vi "motor_log.vi"() -> ()   [LabVIEW 2011]
uses:
  <vilib>/addons/database/Auxilliary.llb/DB Tools Format Datetime String (Time Stamp).vi
  <vilib>/addons/database/Connection.llb/DB Tools Open Connec (String).vi
  <vilib>/addons/database/NI_Database_API.lvlib
  Program Files (x86)/National Instruments/LabVIEW 2011/resource/objmgr/daqmx.rc
panel:
  out "Channels":refnum<k21>[](array[refnum])
  out "decimal integer string":string
  out "Array":dbl[](array[numeric])
  out "Degrees":u32
  out "Boolean 2":bool
  out "Steps":u32
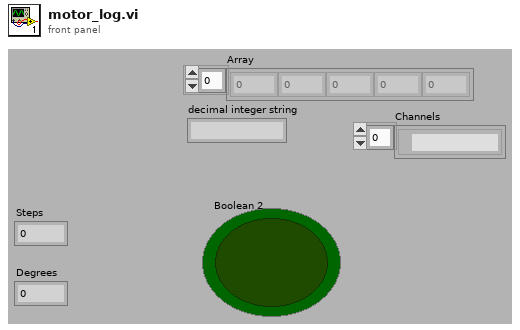
[diagram p1: front panel]
types:
  T1 = typedef "NI_Database_API.lvlib/Conn ObjectReference.ctl" = refnum<k1>
  T2 = cluster{"Array[0]":dbl, "Array[1]":dbl, "Array[2]":dbl, "Array[3]":dbl, "Array[4]":dbl, "Array[5]":dbl, "Array[6]":dbl, "Array[7]":dbl, "Array[8]":dbl}
  T3 = cluster{"date/time string":string, dbl, "Array":cluster{"Array[0]":dbl, "Array[1]":dbl, "Array[2]":dbl, "Array[3]":dbl, "Array[4]":dbl, "Array[5]":dbl, "Array[6]":dbl, "Array[7]":dbl, "Array[8]":dbl}}
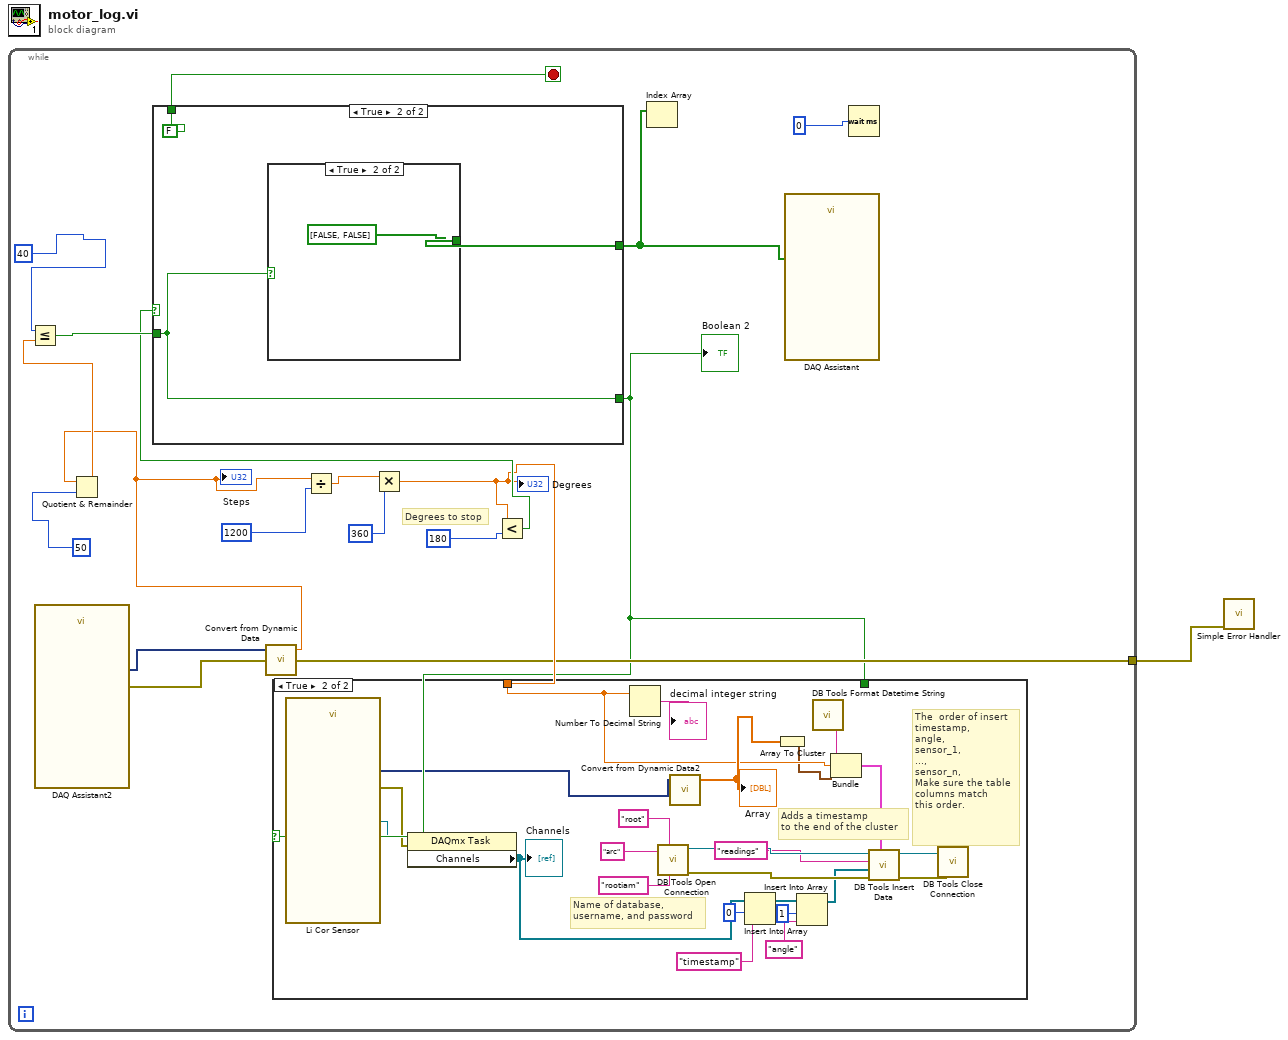
[diagram p0: block diagram]
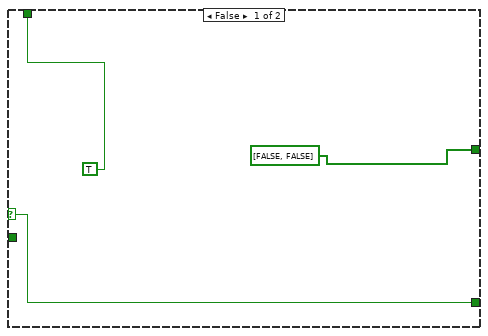
[diagram p3: hidden frame]
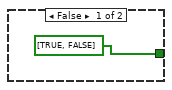
[diagram p4: hidden frame]
diagram:
  n1 = while {
    tunnel: [w5] -> w1
    stop <- w10 stop-if-true
    # "Degrees to stop"
    n2 = call "DAQ Assistant2"() -> ("data"=w6:dynamicdata, "error out"=w5:errorcluster)  [unwired: 16 in, 2 out]
    n3 = call "Convert from Dynamic Data"("Dynamic Data Type"=w6) -> ("Scalar"=w8:dbl)  [unwired: 3 in]
    "Steps" <- w8
    n4 = Quotient & Remainder(x=w8, y=50) -> (x-y*floor(x/y)=w12:dbl)  [unwired: 1 out]
    n5 = Less Or Equal?(x=40, y=w12) -> (x <= y?=w18:bool)
    n6 = Divide(x=w8, y=1200) -> (x/y=w16:dbl)
    n7 = Multiply(x=w16, y=360) -> (x*y=w7:dbl)
    "Degrees" <- w7
    n8 = Less?(x=w7, y=180) -> (x < y?=w11:bool)
    n9 = case shown="True" w11 {
      selector: w11 -> [w45 _]
      tunnel: w18 -> [_ w46]
      tunnel: [w45 w46] -> w2
      tunnel: [TRUE FALSE] -> w10
      tunnel: [bool[] [FALSE, FALSE] w47] -> w4
      frame False {
      }
      frame True {
        n10 = case shown="True" w46 {
          tunnel: [bool[] [TRUE, FALSE] bool[] [FALSE, FALSE]] -> w47
          frame False {
          }
          frame True {
          }
        }
      }
    }
    "Boolean 2" <- w2
    n11 = case shown="True" w2 {
      tunnel: w7 -> [_ w29]
      tunnel: w2 -> [_ _]
      frame False {
      }
      frame True {
        # "The  order of insert\ntimestamp,\nangle,\nsensor_1,\n...,\nsensor_n,\nMake sure the table\ncolumns match \nthis order."
        # "Name of database,\nusername, and password"
        # "Adds a timestamp\nto the end of the cluster"
        n12 = call "Li Cor Sensor"() -> ("task out"=w27:refnum<k21>, "data"=w42:dynamicdata, "error out"=w26:errorcluster)  [unwired: 16 in, 1 out]
        n13 = property class="DAQmx Task"(reference=w27, error in=w26) -> ("Channels"=w25:refnum<k21>[])  [unwired: 2 out]
        "Channels" <- w25
        n14 = Number To Decimal String(number=w29) -> (decimal integer string=→"decimal integer string":string)  [unwired: 1 in]
        n15 = call-poly <vilib>:"DB Tools Open Connection.vi"("password"="rootiam", "userID"="root", "connection information"="arc") -> ("error out"=w39:errorcluster, "connection reference"=w40:T1)  [unwired: 5 in]
        n16 = call "Convert from Dynamic Data2"("Dynamic Data Type"=w42) -> ("Array"=w35:dbl[])  [unwired: 3 in]
        "Array" <- w35
        n17 = Insert Into Array(array=w25, index=0, new element="timestamp") -> (w22:refnum<k21>[])
        n18 = Array To Cluster(array=w35) -> (cluster=w28:T2)
        n19 = Insert Into Array(array=w22, index=1, new element="angle") -> (w19:refnum<k21>[])
        n20 = call-poly <vilib>:"DB Tools Format Datetime String.vi"() -> ("date/time string"=w30:string)  [unwired: 1 in]
        n21 = Bundle("date/time string"=w30, w29, "Array"=w28) -> (w34:T3)  [unwired: 1 in]
        n22 = call <vilib>:"DB Tools Insert Data.vi"("data"=w34, "error in (no error)"=w39, "columns"=w19, "table"="readings", "connection reference"=w40) -> ("error out"=w36:errorcluster, "connection reference out"=w37:T1)  [unwired: 5 in]
        n23 = call <vilib>:"DB Tools Close Connection.vi"("error in (no error)"=w36, "connection reference"=w37) -> ()  [unwired: 5 in, 1 out]
      }
    }
    n24 = Index Array(array=w4) -> ()  [unwired: 1 in, 1 out]
    n25 = call "DAQ Assistant"("data"=w4) -> ()  [unwired: 17 in, 2 out]
    n26 = Wait (ms)(milliseconds to wait=0) -> ()  [unwired: 1 out]
  }
  n27 = call <vilib>:"Simple Error Handler.vi"("error in (no error)"=w1) -> ()  [unwired: 4 in, 5 out]
